vi "loadMSTReleaseForm.vi"() -> ()   [LabVIEW 2012]
uses:
  <vilib>/Utility/NIReport.llb/NI_report.lvclass
  <vilib>/addons/database/Connection.llb/DB Tools Open Connec (Path).vi
  <vilib>/addons/_office/excel.llb/Excel Get Data (str).vi
  <vilib>/addons/database/Connection.llb/Conn Execute.vi
  <vilib>/addons/database/Recordset.llb/Rec Fetch Integer Data (R).vi
  <vilib>/addons/database/Recordset.llb/Rec Destroy - Connection.vi
  <vilib>/Utility/NIReport.llb/Excel/NI_Excel.lvclass
  <vilib>/addons/_office/NI_ReportGenerationToolkit.lvlib
  <vilib>/addons/database/NI_Database_API.lvlib
panel:
  out "error out 2":errorcluster
  out "error out":errorcluster
  out "appended path":path
  out "String":string
  out "concatenated string":string
  out "error out 4":errorcluster
  out "date/time string":string
  out "x+y":dbl
  out "Product":string
  out "Temp":string
  out "TestTime":string
  out "TestProgram":string
  out "PCB":string
  in  "start (0, 0)":cluster{"start row":i32, "start column":i32}
  out "row":i32
  in  "path":path=path "O:/Monitor/Recipe/MST"
  out "filenames":string[](array[string])
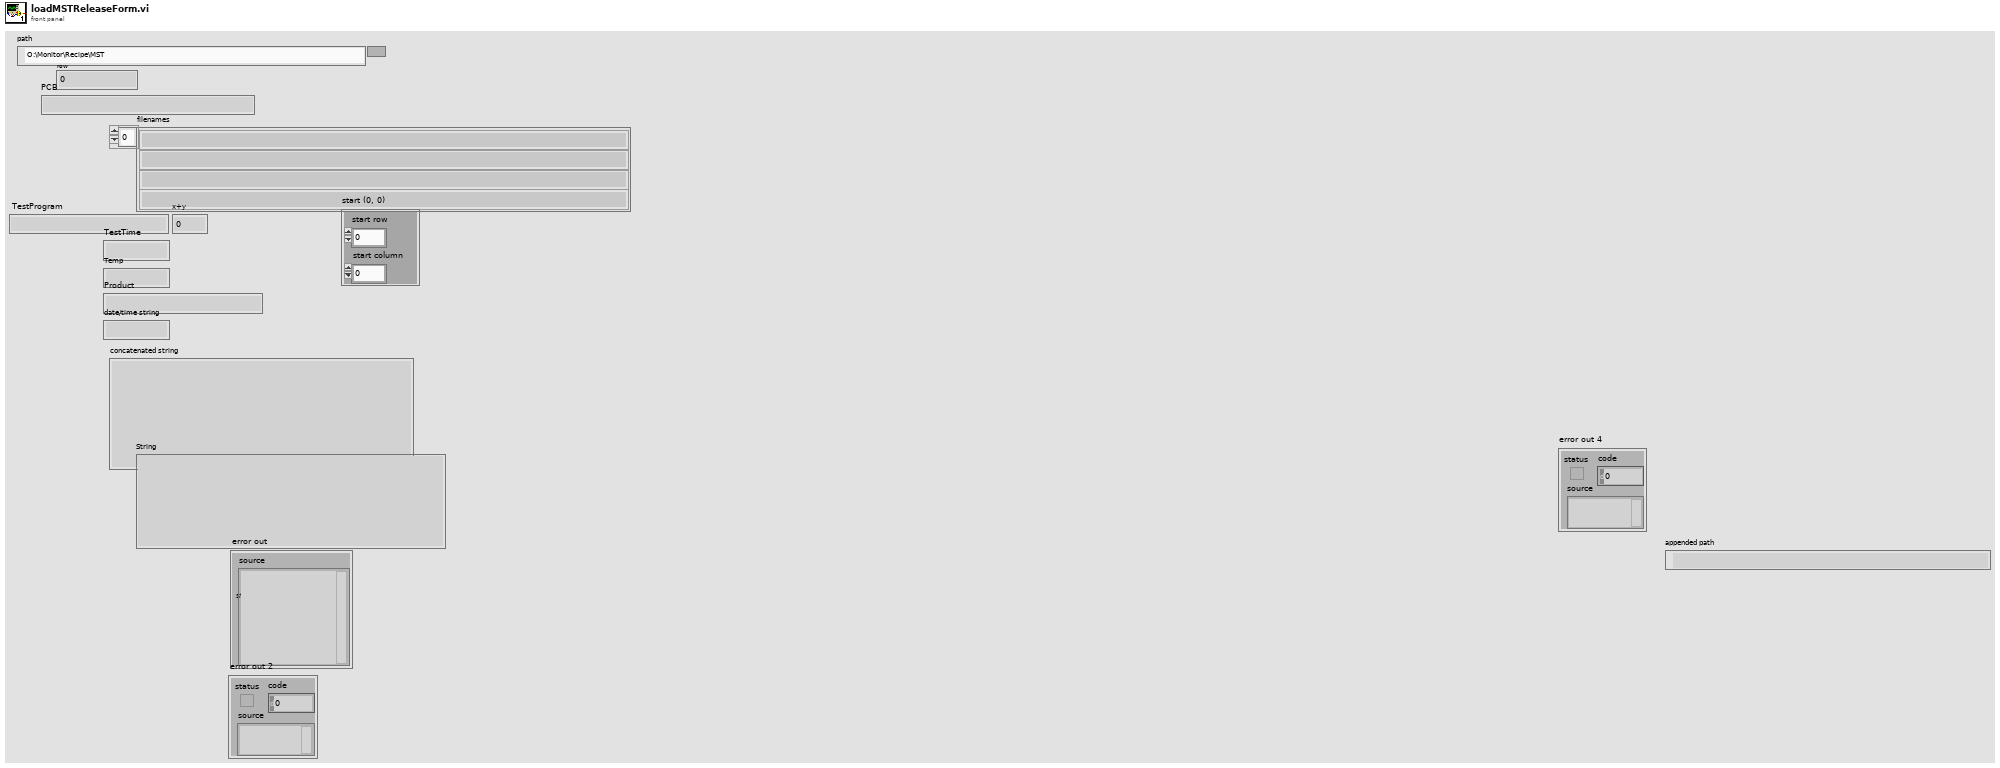
[diagram p1: front panel]
types:
  T1 = enum16{"Standard Report", "HTML", "Word", "Excel"}
  T2 = typedef "NI_Database_API.lvlib/Conn ObjectReference.ctl" = refnum<k1>
  T3 = typedef "NI_Database_API.lvlib/Rec ObjectReference.ctl" = refnum<k1>
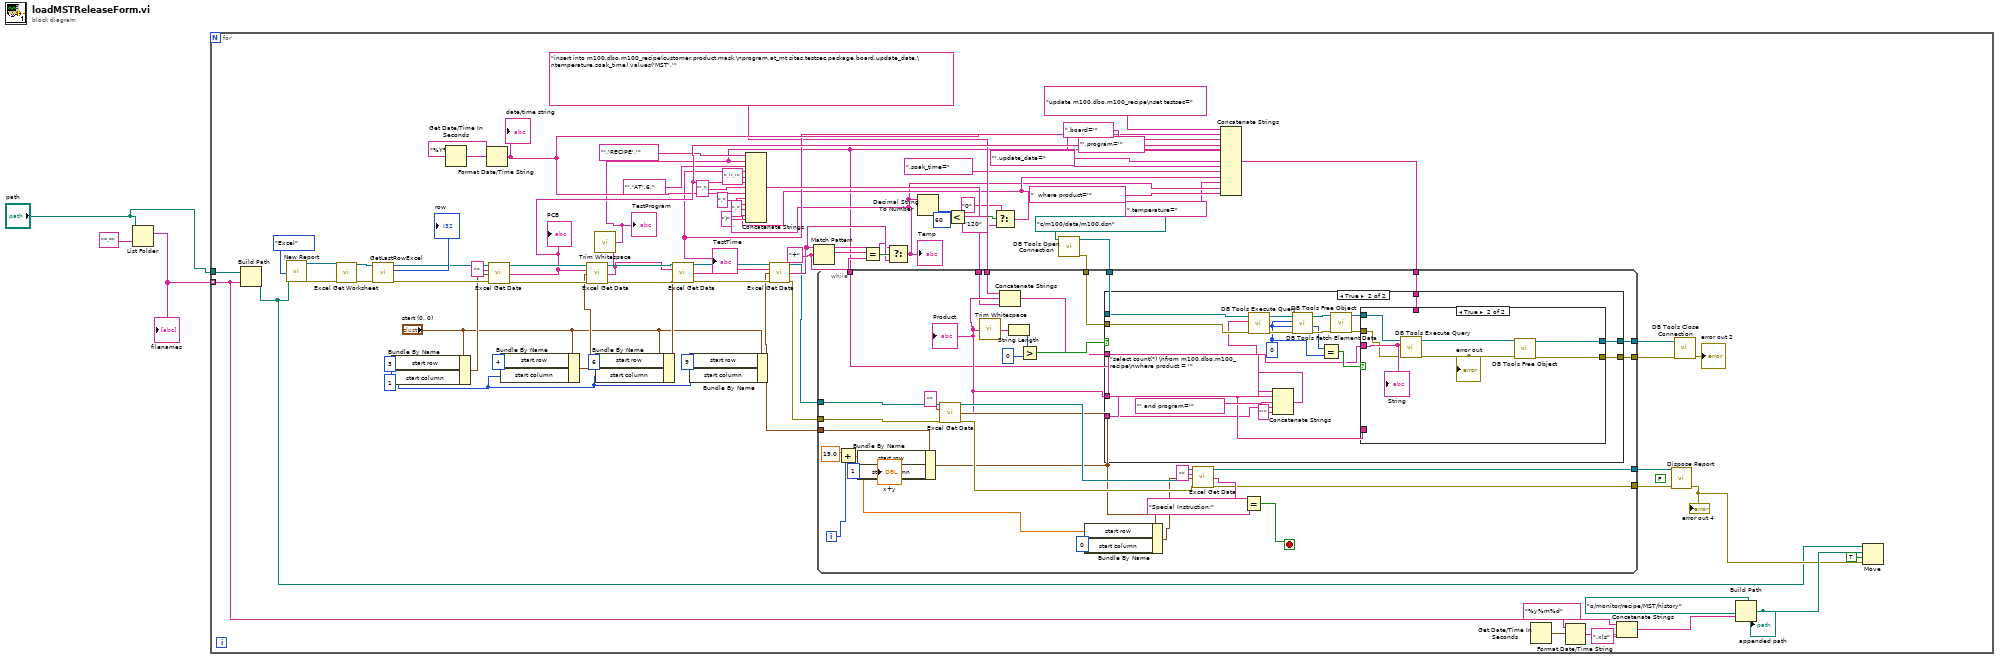
[diagram p0: block diagram]
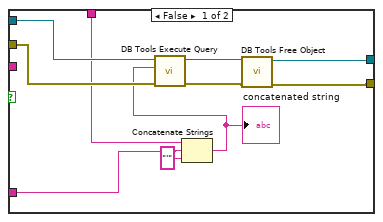
[diagram p3: hidden frame]
diagram:
  n1 = List Folder(path="path", pattern="*.*") -> (filenames=w1:string[])  [unwired: 2 in, 3 out]
  "filenames" <- w1
  n2 = for {
    tunnel: "path" -> [w81]
    tunnel: w1 -> [w23] mode=indexing
    (unwired) FALSE ("save changes? (F)")
    w60 = "+" ("regular expression")
    w66 = 1 ("start column")
    n3 = Build Path(base path=w81, name or relative path=w23) -> (appended path=w24:path)
    n4 = call <vilib>:"New Report.vi"("report type"=T1."Excel" ("Report Type"), "template (empty)"=w24) -> ("report out"=w85:refnum<class "NI_report.lvclass">, "error out"=w84:errorcluster)  [unwired: 12 in]
    n5 = call <vilib>:"Excel Get Worksheet.vi"("report in"=w85, "error in (no error)"=w84) -> ("report out"=w83:refnum<class "NI_report.lvclass">, "error out"=w82:errorcluster)  [unwired: 12 in]
    n6 = call "GetLastRowExcel.vi"("error in (no error)"=w82, "report in"=w83) -> ("error out"=w79:errorcluster, "row"=→"row":i32, "report out"=w78:refnum<class "NI_report.lvclass">)  [unwired: 7 in]
    n7 = Bundle By Name(cluster="start (0, 0)", "start row"=3, "start column"=w66) -> (w77:cluster{"start row":i32, "start column":i32})
    n8 = Get Date/Time In Seconds() -> (seconds since 1Jan1904=w49:timestamp)
    n9 = Format Date/Time String(time format string (%c)="%Y%m%d", seconds (now)=w49) -> (date/time string=w35:string)  [unwired: 1 in]
    "date/time string" <- w35
    n10 = call-poly <vilib>:"Excel Get Data.vi"("report in"=w78, "data type"="", "start (0, 0)"=w77, "error in (no error)"=w79) -> ("report out"=w73:refnum<class "NI_report.lvclass">, "data"=w38:string, "error out"=w74:errorcluster)  [unwired: 9 in]
    "PCB" <- w38
    n11 = Bundle By Name(cluster="start (0, 0)", "start row"=4, "start column"=w66) -> (w71:cluster{"start row":i32, "start column":i32})
    n12 = call-poly <vilib>:"Excel Get Data.vi"("report in"=w73, "data type"=w38, "start (0, 0)"=w71, "error in (no error)"=w74) -> ("report out"=w70:refnum<class "NI_report.lvclass">, "data"=w5:string, "error out"=w69:errorcluster)  [unwired: 9 in]
    n13 = call <vilib>:"Trim Whitespace.vi"("string"=w5) -> ("trimmed string"=w4:string)  [unwired: 1 in]
    "TestProgram" <- w4
    n14 = Bundle By Name(cluster="start (0, 0)", "start row"=6, "start column"=w66) -> (w67:cluster{"start row":i32, "start column":i32})
    n15 = call-poly <vilib>:"Excel Get Data.vi"("report in"=w70, "data type"=w5, "start (0, 0)"=w67, "error in (no error)"=w69) -> ("report out"=w63:refnum<class "NI_report.lvclass">, "data"=w19:string, "error out"=w64:errorcluster)  [unwired: 9 in]
    "TestTime" <- w19
    n16 = Bundle By Name(cluster="start (0, 0)", "start row"=9, "start column"=w66) -> (w54:cluster{"start row":i32, "start column":i32})
    n17 = call-poly <vilib>:"Excel Get Data.vi"("report in"=w63, "data type"=w19, "start (0, 0)"=w54, "error in (no error)"=w64) -> ("report out"=w56:refnum<class "NI_report.lvclass">, "data"=w58:string, "error out"=w55:errorcluster)  [unwired: 9 in]
    n18 = Match Pattern(string=w58, regular expression=w60) -> (before substring=w57:string, match substring=w61:string)  [unwired: 1 in, 2 out]
    n19 = Equal?(x=w61, y=w60) -> (x = y?=w59:bool)
    n20 = Select(t=w57, s=w59, f=w58) -> (s? t:f=w7:string)
    "Temp" <- w7
    n21 = Decimal String To Number(string=w7) -> (number=w17:i32)  [unwired: 2 in, 1 out]
    n22 = Less?(x=w17, y=60) -> (x < y?=w15:bool)
    n23 = Select(t="0", s=w15, f="120") -> (s? t:f=w8:string)
    n24 = Concatenate Strings("','RECIPE','" ("string"), w4, "','AT',6," ("string"), w19, ",'','" ("string"), w38, "'," ("string"), w35, "," ("string"), w7, "," ("string"), w8, ")" ("string")) -> (w45:string)
    n25 = call-poly <vilib>:"DB Tools Open Connection.vi"("connection information"=path "c:/m100/data/m100.dsn") -> ("error out"=w52:errorcluster, "connection reference"=w53:T2)  [unwired: 7 in]
    n26 = Concatenate Strings("update m100.dbo.m100_recipe\nset testsec=", w19, ",board='" ("string"), w38, "',program='" ("string"), w4, "',update_date=" ("string"), w35, ",soak_time=" ("string"), w8, ",temperature=" ("string"), w7, "  where product='" ("string")) -> (w34:string)
    n27 = while {
      tunnel: w56 -> [w119]
      tunnel: w55 -> [w118]
      tunnel: w54 -> [w117]
      tunnel: w53 -> [w98]
      tunnel: w52 -> [w97]
      tunnel: "insert into m100.dbo.m100_recipe(customer,product,mask,\nprogram,at_mt,sites,testsec,package,board,update_date,\ntemperature,soak_time) values('MST','" ("string") -> [w96]
      tunnel: w45 -> [w94]
      tunnel: [w92] -> w44
      tunnel: [w91] -> w43
      tunnel: [w90] -> w42
      tunnel: [w89] -> w41
      tunnel: w34 -> [w88]
      tunnel: w4 -> [w87]
      i -> [w110]
      stop <- w100 stop-if-true
      n28 = Add(x=19.0, y=w110) -> (x+y=w109:dbl)
      "x+y" <- w109
      n29 = Bundle By Name(cluster=w117, "start row"=w109, "start column"=1) -> (w104:cluster{"start row":i32, "start column":i32})
      n30 = call-poly <vilib>:"Excel Get Data.vi"("report in"=w119, "data type"="", "start (0, 0)"=w104, "error in (no error)"=w118) -> ("report out"=w106:refnum<class "NI_report.lvclass">, "data"=w95:string, "error out"=w107:errorcluster)  [unwired: 9 in]
      "Product" <- w95
      n31 = call <vilib>:"Trim Whitespace.vi"("string"=w95) -> ("trimmed string"=w114:string)  [unwired: 1 in]
      n32 = Concatenate Strings(w96, w95, w94) -> (w93:string)
      n33 = String Length(string=w114) -> (length=w113:i32)
      n34 = Greater?(x=w113, y=0) -> (0:w99:bool)
      n35 = Bundle By Name(cluster=w104, "start row"=w109, "start column"=0) -> (w105:cluster{"start row":i32, "start column":i32})
      n36 = case shown="True" w99 {
        tunnel: w98 -> [w121 w142]
        tunnel: w97 -> [w120 w141]
        tunnel: w95 -> [_ w124]
        tunnel: w93 -> [_ w126]
        tunnel: [w121 w128] -> w92
        tunnel: [w120 w127] -> w91
        tunnel: w88 -> [_ w125]
        tunnel: w87 -> [_ w123]
        frame False {
        }
        frame True {
          w132 = 0
          n37 = Concatenate Strings("select count(*) \nfrom m100.dbo.m100_recipe\nwhere product = '" ("string"), w124, "' and program='" ("string"), w123, "'" ("string")) -> (w138:string)
          n38 = call-poly <vilib>:"DB Tools Execute Query.vi"("error in (no error)"=w141, "SQL query"=w138, "connection reference"=w142) -> ("error out"=w136:errorcluster, "recordset reference"=w137:T3)  [unwired: 5 in]
          n39 = call-poly <vilib>:"DB Tools Fetch Element Data.vi"("error in (no error)"=w136, "type"=w132, "column index"=w132, "recordset reference"=w137) -> ("error out"=w134:errorcluster, "data"=w133:i32, "recordset reference out"=w135:T3)  [unwired: 3 in]
          n40 = Equal?(x=w133, y=w132) -> (x = y?=w131:bool)
          n41 = call-poly <vilib>:"DB Tools Free Object.vi"("error in (no error)"=w134, "recordset reference"=w135) -> ("error out"=w129:errorcluster, "connection reference"=w130:T2)  [unwired: 8 in]
          n42 = case shown="True" w131 {
            tunnel: w126 -> [_ w159]
            tunnel: w130 -> [w152 w158]
            tunnel: w129 -> [w151 w157]
            tunnel: [w148 w154] -> w128
            tunnel: [w147 w153] -> w127
            tunnel: w125 -> [w146 _]
            tunnel: w124 -> [w145 _]
            frame False {
              n43 = Concatenate Strings(w146, w145, "'" ("string")) -> (w143:string)
              "concatenated string" <- w143
              n44 = call-poly <vilib>:"DB Tools Execute Query.vi"("error in (no error)"=w151, "SQL query"=w143, "connection reference"=w152) -> ("error out"=w149:errorcluster, "recordset reference"=w150:T3)  [unwired: 5 in]
              n45 = call-poly <vilib>:"DB Tools Free Object.vi"("error in (no error)"=w149, "recordset reference"=w150) -> ("error out"=w147:errorcluster, "connection reference"=w148:T2)  [unwired: 8 in]
            }
            frame True {
              n46 = call-poly <vilib>:"DB Tools Execute Query.vi"("error in (no error)"=w157, "SQL query"=w159, "connection reference"=w158) -> ("error out"=w156:errorcluster, "recordset reference"=w155:T3)  [unwired: 5 in]
              "error out" <- w156
              n47 = call-poly <vilib>:"DB Tools Free Object.vi"("error in (no error)"=w156, "recordset reference"=w155) -> ("error out"=w153:errorcluster, "connection reference"=w154:T2)  [unwired: 8 in]
              "String" <- w159
            }
          }
        }
      }
      n48 = call-poly <vilib>:"Excel Get Data.vi"("report in"=w106, "data type"="", "start (0, 0)"=w105, "error in (no error)"=w107) -> ("report out"=w90:refnum<class "NI_report.lvclass">, "data"=w102:string, "error out"=w89:errorcluster)  [unwired: 9 in]
      n49 = Equal?(x=w102, y="Special Instruction:") -> (x = y?=w100:bool)
    }
    n50 = Get Date/Time In Seconds() -> (seconds since 1Jan1904=w31:timestamp)
    n51 = Format Date/Time String(time format string (%c)="%y%m%d", seconds (now)=w31) -> (date/time string=w29:string)  [unwired: 1 in]
    n52 = Concatenate Strings(w23, w29, ".xls" ("string")) -> (w32:string)
    n53 = call-dynamic "Dispose Report.vi"("report in"=w42, "error in (no error)"=w41) -> ("error out"=w25:errorcluster)  [unwired: 13 in]
    "error out 4" <- w25
    n54 = call <vilib>:"DB Tools Close Connection.vi"("error in (no error)"=w43, "connection reference"=w44) -> ("error out"=→"error out 2":errorcluster)  [unwired: 5 in]
    n55 = Build Path(base path=path "o:/monitor/recipe/MST/history", name or relative path=w32) -> (appended path=w27:path)
    "appended path" <- w27
    n56 = Move(source path=w24, error in=w25, 9:TRUE ("overwrite (F)"), 10:w27) -> ()  [unwired: 1 in, 3 out]
  }
